vi "serpenbot_DDPG_learing_parallel.vi"() -> ()   [LabVIEW 2020]
uses:
  <vilib>/Analysis/Matrix/Datatypes/RealMatrix.ctl
  <vilib>/Analysis/Matrix/NI_Matrix.lvlib
  <vilib>/Analysis/NI_AALBase.lvlib
  <vilib>/Analysis/baseanly.llb/Real A x B.vi
  <vilib>/Analysis/NI_AALPro.lvlib
  <vilib>/Analysis/Matrix/Numeric/Conversions/Array To Matrix - RA.vi
  <vilib>/Analysis/Matrix/Numeric/Subtract/Subtract - RM,RM.vi
  <vilib>/Analysis/_algsub.llb/Real PseudoInverse Matrix.vi
panel:
  out "error out Y":errorcluster
  out "error out X":errorcluster
  out "laser control value":dbl[](array[numeric])
  out "current y":dbl
  out "current x":dbl
  out "control_loop_time":u32
  in  "stop":bool
  in  "Logging":bool caption="Enable"
  in  "k":T1
  in  "Diode Current\nSetting":dbl=3.0
  in  "Laser Repetition\nFrequency":i32=50000
  in  "VISA resource name":refnum<visa-resource-name>="COM14"
  in  "baud rate (9600)":u32=9600
  out "error out":errorcluster
  out "Identification system 1":string
  out "Conn. axes system 1":string[](array[string])
  out "Identification system 2":string
  out "Conn. axes system  2":string[](array[string])
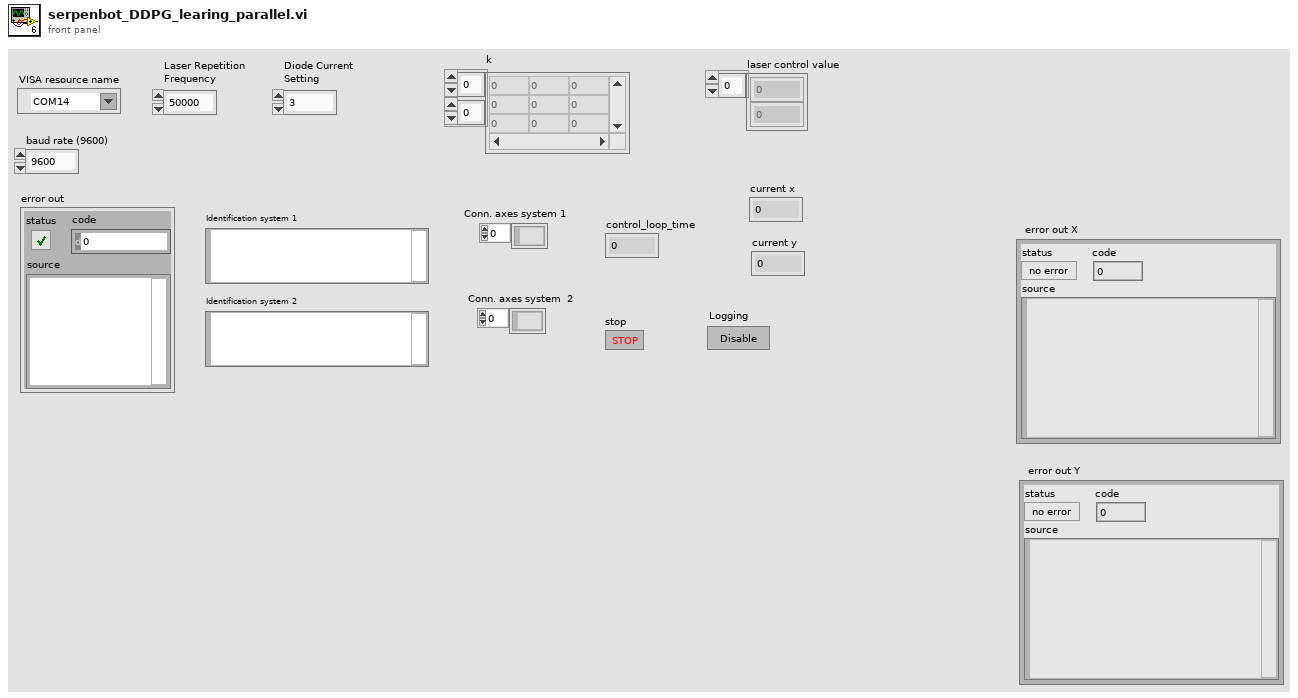
[diagram p1: front panel]
types:
  T1 = typedef "NI_Matrix.lvlib/RealMatrix.ctl" = dbl[][]
  T2 = cluster{"RS232 settings":cluster{"Portnumber":i32, "Baudrate":u16}, "USB settings":cluster{"S/N":string, "USB Search?":bool}, "TCP/IP settings":cluster{"Host address/name":string, "Port":i32, "Board":i32, "TCP/IP Search?":bool}}
  T3 = cluster{"Check FRF?":bool, "Referencing mode":enum16{"FRF (-> FNL)", "FRF", "FNL", "FPL", "RON OFF"}[]}
  T4 = cluster{"Force?":bool, "Dialog?":bool, "Stages":string[]}
  T5 = cluster{"Position":cluster{"x":sgl, "y":sgl}, "Angle":sgl, "Scale":sgl, "Score":sgl, "Bounding Box":cluster{"x":sgl, "y":sgl}[]}[]
  T6 = cluster{"[0]":cluster{"Position":cluster{"x":sgl, "y":sgl}, "Angle":sgl, "Scale":sgl, "Score":sgl, "Bounding Box":cluster{"x":sgl, "y":sgl}[]}, "[1]":cluster{"Position":cluster{"x":sgl, "y":sgl}, "Angle":sgl, "Scale":sgl, "Score":sgl, "Bounding Box":cluster{"x":sgl, "y":sgl}[]}, "[2]":cluster{"Position":cluster{"x":sgl, "y":sgl}, "Angle":sgl, "Scale":sgl, "Score":sgl, "Bounding Box":cluster{"x":sgl, "y":sgl}[]}, "[3]":cluster{"Position":cluster{"x":sgl, "y":sgl}, "Angle":sgl, "Scale":sgl, "Score":sgl, "Bounding Box":cluster{"x":sgl, "y":sgl}[]}, "[4]":cluster{"Position":cluster{"x":sgl, "y":sgl}, "Angle":sgl, "Scale":sgl, "Score":sgl, "Bounding Box":cluster{"x":sgl, "y":sgl}[]}, "[5]":cluster{"Position":cluster{"x":sgl, "y":sgl}, "Angle":sgl, "Scale":sgl, "Score":sgl, "Bounding Box":cluster{"x":sgl, "y":sgl}[]}, "[6]":cluster{"Position":cluster{"x":sgl, "y":sgl}, "Angle":sgl, "Scale":sgl, "Score":sgl, "Bounding Box":cluster{"x":sgl, "y":sgl}[]}, "[7]":cluster{"Position":cluster{"x":sgl, "y":sgl}, "Angle":sgl, "Scale":sgl, "Score":sgl, "Bounding Box":cluster{"x":sgl, "y":sgl}[]}, "[8]":cluster{"Position":cluster{"x":sgl, "y":sgl}, "Angle":sgl, "Scale":sgl, "Score":sgl, "Bounding Box":cluster{"x":sgl, "y":sgl}[]}}
  T7 = cluster{"Position":cluster{"x":sgl, "y":sgl}, "Angle":sgl, "Scale":sgl, "Score":sgl, "Bounding Box":cluster{"x":sgl, "y":sgl}[]}
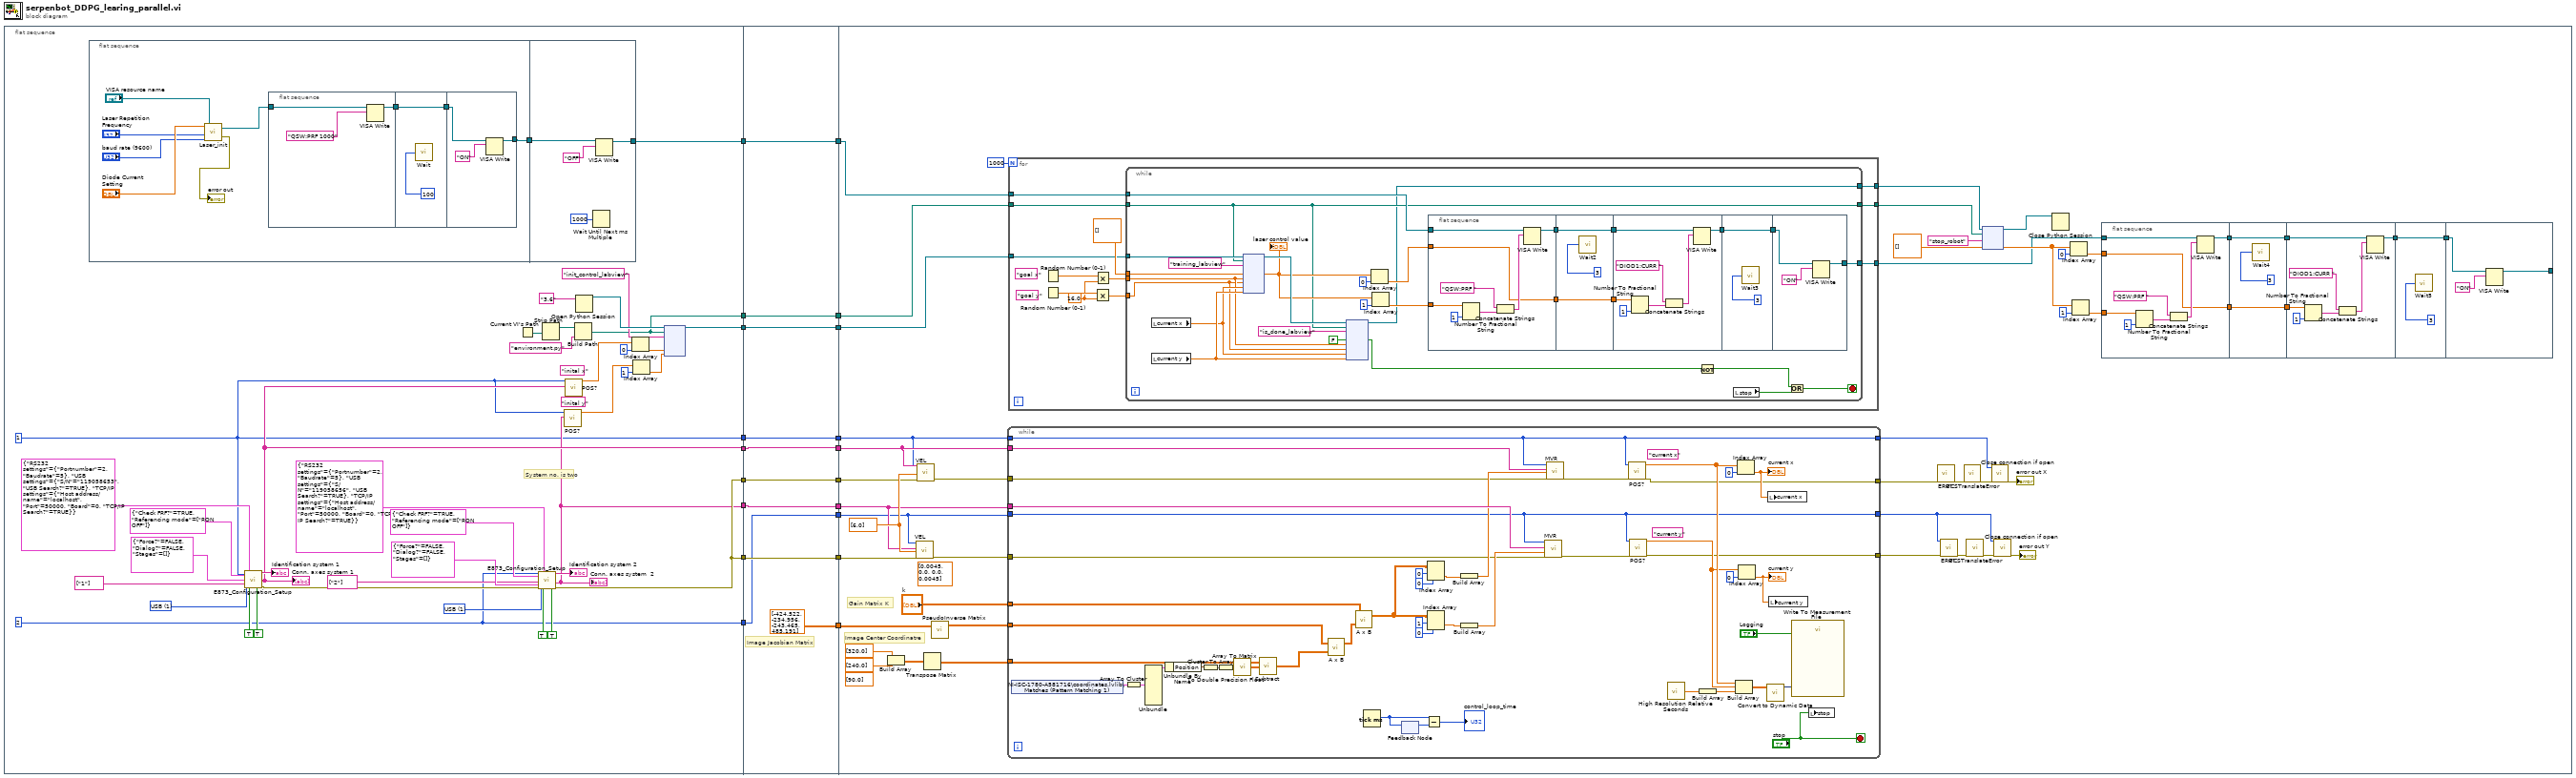
[diagram p0: block diagram]
diagram:
  n1 = flat-sequence {
    tunnel: [w56] -> w19
    tunnel: [w26] -> w18
    tunnel: [w28] -> w17
    tunnel: [w37] -> w16
    tunnel: [w27] -> w15
    tunnel: [w38] -> w14
    tunnel: [w37] -> w13
    tunnel: [w30] -> w12
    tunnel: [w29] -> w11
    tunnel: w19 -> [w88]
    tunnel: [w88] -> w10
    tunnel: w18 -> [w87]
    tunnel: w17 -> [w86]
    tunnel: w16 -> [w85]
    tunnel: w15 -> [w84]
    tunnel: w14 -> [w82]
    tunnel: [w87] -> w9
    tunnel: [w86] -> w8
    tunnel: [w85] -> w7
    tunnel: [w84] -> w6
    tunnel: w13 -> [w83]
    tunnel: [w83] -> w5
    tunnel: [w82] -> w4
    tunnel: [T1 [[-424.522, -234.956], [-243.465, 485.191]] ("J_init 2")] -> w3
    tunnel: w12 -> [w80]
    tunnel: w11 -> [w79]
    tunnel: [w80] -> w2
    tunnel: [w79] -> w1
    tunnel: w10 -> [w103]
    tunnel: w9 -> [w121]
    tunnel: w8 -> [w128]
    tunnel: w7 -> [w131]
    tunnel: w6 -> [w126]
    tunnel: w5 -> [w130]
    tunnel: w4 -> [w120]
    tunnel: w3 -> [w129]
    tunnel: w2 -> [w105]
    tunnel: w1 -> [w104]
    frame #0 {
      (unwired) "inital y"
      (unwired) "inital x"
      w41 = u16 1 items=["RS232", "USB", "TCP/IP"] ("Interface")
      w44 = u16 1 items=["RS232", "USB", "TCP/IP"] ("Interface")
      w38 = 2 ("System no.")
      w26 = 1 ("System no.")
      # "System no. is two"
      n2 = flat-sequence {
        tunnel: [w58] -> w57
        tunnel: w57 -> [w76]
        tunnel: [w75] -> w56
        frame #0 {
          n3 = call "Laser_init.vi"("baud rate (9600)"="baud rate (9600)", "Laser Repetition\nFrequency"="Laser Repetition\nFrequency", "VISA resource name"="VISA resource name", "Diode Current\nSetting"="Diode Current\nSetting") -> ("error out"=→"error out":errorcluster, "VISA Refnum out"=w59:refnum<visa-resource-name>)
          n4 = flat-sequence {
            tunnel: w59 -> [w69]
            tunnel: [w68] -> w66
            tunnel: w66 -> [w71]
            tunnel: [w71] -> w65
            tunnel: w65 -> [w72]
            tunnel: [w73] -> w58
            frame #0 {
              n5 = VISA Write(VISA resource name=w69, write buffer="QSW:PRF 1000" ("string")) -> (VISA resource name out=w68:refnum<visa-resource-name>)  [unwired: 1 in, 2 out]
            }
            frame #1 {
              n6 = call "Wait"("Count(mSec)"=u32 100) -> ()  [unwired: 1 out]
            }
            frame #2 {
              n7 = VISA Write(VISA resource name=w72, write buffer="ON") -> (VISA resource name out=w73:refnum<visa-resource-name>)  [unwired: 1 in, 2 out]
            }
          }
        }
        frame #1 {
          n8 = Wait Until Next ms Multiple(millisecond multiple=u32 1000) -> ()  [unwired: 1 out]
          n9 = VISA Write(VISA resource name=w76, write buffer="OFF") -> (VISA resource name out=w75:refnum<visa-resource-name>)  [unwired: 1 in, 2 out]
        }
      }
      n10 = call "E873_Configuration_Setup.vi"("System no."=w26, "Referencing"=T3 {"Check FRF?"=TRUE, "Referencing mode"=[enum."RON OFF"]}, "Interface"=w44, "All axes?"=TRUE, "Axes to move"=string[] ["1"], "Interface settings"=T2 {"RS232 settings"={"Portnumber"=2, "Baudrate"=5}, "USB settings"={"S/N"="119058653", "USB Search?"=TRUE}, "TCP/IP settings"={"Host address/name"="localhost", "Port"=50000, "Board"=0, "TCP/IP Search?"=TRUE}}, "Stage selection"=T4 {"Force?"=FALSE, "Dialog?"=FALSE, "Stages"=[]}, "Switch servo on?"=TRUE ("Use dialog to define\nconnected stages?")) -> ("Identification"=→"Identification system 1":string, "Conn. \nAxes"=w28:string[], "error out"=w53:errorcluster)  [unwired: 4 in, 5 out]
      "Conn. axes system 1" <- w28
      n11 = Current VI's Path() -> (path=w36:path)
      n12 = call "E873_Configuration_Setup.vi"("System no."=w38, "Referencing"=T3 {"Check FRF?"=TRUE, "Referencing mode"=[enum."RON OFF"]}, "Interface"=w41, "All axes?"=TRUE, "Axes to move"=string[] ["2"], "error in"=w53, "Interface settings"=T2 {"RS232 settings"={"Portnumber"=2, "Baudrate"=5}, "USB settings"={"S/N"="119058656", "USB Search?"=TRUE}, "TCP/IP settings"={"Host address/name"="localhost", "Port"=50000, "Board"=0, "TCP/IP Search?"=TRUE}}, "Stage selection"=T4 {"Force?"=FALSE, "Dialog?"=FALSE, "Stages"=[]}, "Switch servo on?"=TRUE ("Use dialog to define\nconnected stages?")) -> ("Identification"=→"Identification system 2":string, "Conn. \nAxes"=w27:string[], "error out"=w37:errorcluster)  [unwired: 3 in, 5 out]
      "Conn. axes system  2" <- w27
      n13 = Strip Path(path=w36) -> (stripped path=w35:path)  [unwired: 1 out]
      n14 = call "POS?.vi"("System no."=w26, "Axes to query"=w27) -> ("Position"=w20:dbl[])  [unwired: 3 in, 14 out]
      n15 = call "POS?.vi"("System no."=w26, "Axes to query"=w28) -> ("Position"=w23:dbl[])  [unwired: 3 in, 14 out]
      n16 = Build Path(base path=w35, name or relative path="environment.py") -> (appended path=w30:path)
      n17 = Open Python Session(python version="3.6" ("Python version")) -> (session out=w32:refnum<k35>)  [unwired: 2 in, 1 out]
      n18 = Index Array(array=w23, index=0) -> (element=w24:dbl)
      n19 = Index Array(array=w20, index=1) -> (element=w21:dbl)
      n20 = node(w32, w30, "init_control_labview" ("function name"), w24, w21) -> (w29:refnum<k35>)  [unwired: 5 in, 3 out]
    }
    frame #1 {
      # "Image Jacobian Matrix"
    }
    frame #2 {
      w132 = dbl[] [6.0] ("Velocity values")
      (unwired) T1 [[0.0045, 0.0], [0.0, 0.0045]] ("J_init 2")
      (unwired) dbl[] [90.0] ("element")
      # "Gain Matrix K"
      # "Image Center Coordinatre"
      n21 = Build Array(dbl[] [320.0] ("element"), dbl[] [240.0] ("element")) -> (w133:T1)
      n22 = call "VEL.vi"("System no."=w120, "Axes to set"=w126, "Velocity values"=w132, "error in"=w130) -> ("error out"=w125:errorcluster)  [unwired: 2 in, 13 out]
      n23 = call "VEL.vi"("System no."=w121, "Axes to set"=w128, "Velocity values"=w132, "error in"=w131) -> ("error out"=w127:errorcluster)  [unwired: 2 in, 13 out]
      n24 = Transpose Matrix(1:w133) -> (0:w122:T1)
      n25 = call-poly <vilib>:"PseudoInverse Matrix.vi"("Input Matrix"=w129) -> ("PseudoInverse Matrix"=w123:T1)  [unwired: 1 in, 1 out]
      n26 = while {
        tunnel: w125 -> [w227]
        tunnel: w120 -> [w201]
        tunnel: w126 -> [w245]
        tunnel: w127 -> [w228]
        tunnel: w128 -> [w244]
        tunnel: w121 -> [w203]
        tunnel: w123 -> [w233]
        tunnel: "k" -> [w232]
        tunnel: w122 -> [w231]
        tunnel: [w203] -> w92
        tunnel: [w202] -> w91
        tunnel: [w201] -> w90
        tunnel: [w200] -> w89
        stop <- "stop" stop-if-true
        (unwired) "current y"
        (unwired) "current x"
        n27 = shared-variable "NI-ISC-1780-A581716\\coordinates.lvlib\\Matches (Pattern Matching 1)"() -> (w220:T5)  [unwired: 1 in, 1 out]
        n28 = Array To Cluster(array=w220) -> (cluster=w221:T6)
        n29 = Unbundle(w221) -> ("[0]"=w222:T7)  [unwired: 8 out]
        n30 = Unbundle By Name(w222) -> ("Position"=w223:cluster{"x":sgl, "y":sgl})
        n31 = Cluster To Array(cluster=w223) -> (array=w224:sgl[])
        n32 = To Double Precision Float(number=w224) -> (double precision float=w225:dbl[])
        n33 = call-poly <vilib>:"Array To Matrix.vi"("Real 1D Array"=w225) -> ("Real Matrix (Column Vector)"=w219:T1)
        n34 = call-poly <vilib>:"Subtract.vi"("Real Matrix B"=w219, "Real Matrix A"=w231) -> ("A - B"=w239:T1)
        n35 = call-poly <vilib>:"A x B.vi"("B"=w239, "A"=w233) -> ("A x B"=w237:T1)  [unwired: 1 out]
        n36 = call-poly <vilib>:"A x B.vi"("B"=w237, "A"=w232) -> ("A x B"=w238:T1)  [unwired: 1 out]
        n37 = Tick Count (ms)() -> (millisecond timer value=w211:u32)
        n38 = feedback #1() -> (w234:u32)  [unwired: 1 in]
        n39 = feedback-in #1(w211) -> ()
        n40 = Subtract(x=w211, y=w234) -> (x-y=→"control_loop_time":u32)
        n41 = Index Array(array=w238, index (row)=0, index (col)=0) -> (element=w230:dbl)
        n42 = Index Array(array=w238, index (row)=1, index (col)=0) -> (element=w229:dbl)
        n43 = Build Array(w230) -> (w236:dbl[])
        n44 = Build Array(w229) -> (w235:dbl[])
        n45 = call "MVR.vi"("System no."=w201, "Axes to move"=w245, "Position values"=w235, "error in"=w227) -> ("error out"=w212:errorcluster)  [unwired: 1 in, 14 out]
        n46 = call "MVR.vi"("System no."=w203, "Axes to move"=w244, "Position values"=w236, "error in"=w228) -> ("error out"=w213:errorcluster)  [unwired: 1 in, 14 out]
        n47 = call "POS?.vi"("System no."=w203, "error in"=w213) -> ("Position"=w210:dbl[], "error out"=w202:errorcluster)  [unwired: 3 in, 13 out]
        n48 = call "POS?.vi"("System no."=w201, "error in"=w212) -> ("Position"=w208:dbl[], "error out"=w200:errorcluster)  [unwired: 3 in, 13 out]
        n49 = call <vilib>:"High Resolution Relative Seconds.vi"() -> ("relative seconds"=w215:dbl)
        n50 = Build Array(w215) -> (w214:dbl[])
        n51 = Build Array(w210, w208, w214) -> (w217:dbl[][])
        n52 = Index Array(array=w210, index=0) -> (element=w206:dbl)
        "current x" <- w206
        n53 = Index Array(array=w208, index=0) -> (element=w205:dbl)
        "current y" <- w205
        n54 = call "Convert to Dynamic Data"("2D Array"=w217) -> ("Dynamic Data Type"=w216:dynamicdata)  [unwired: 3 in]
        n55 = local write "current x"(w206) -> ()
        n56 = local write "current y"(w205) -> ()
        n57 = call "Write To Measurement File"("Signals"=w216, "Enable"="Logging") -> ()  [unwired: 15 in, 3 out]
        n58 = local write "stop"("stop") -> ()
      }
      n59 = for {
        N: 1000 -> [_]
        tunnel: w105 -> [w141]
        tunnel: w104 -> [w140]
        tunnel: w103 -> [w139]
        tunnel: [w138] -> w101
        tunnel: [w137] -> w100
        tunnel: [w136] -> w99
        w145 = 16.0
        (unwired) "goal y"
        (unwired) "goal x"
        n60 = Random Number (0-1)() -> (number: 0 to 1=w147:dbl)
        n61 = Random Number (0-1)() -> (number: 0 to 1=w146:dbl)
        n62 = Multiply(x=w146, y=w145) -> (x*y=w142:dbl)
        n63 = Multiply(x=w147, y=w145) -> (x*y=w143:dbl)
        n64 = while {
          tunnel: dbl[] [] -> [w161]
          tunnel: w143 -> [w158]
          tunnel: w142 -> [w157]
          tunnel: w141 -> [w154]
          tunnel: w140 -> [w156]
          tunnel: w139 -> [w155]
          tunnel: [w154] -> w138
          tunnel: [w153] -> w137
          tunnel: [w148] -> w136
          stop <- w151 stop-if-true
          n65 = local read "current x"() -> (w159:dbl)
          n66 = local read "current y"() -> (w160:dbl)
          n67 = node(w156, w154, "training_labview" ("function name"), w161, w158, w157, w159, w160) -> (w169:refnum<k35>, w163:dbl[])  [unwired: 5 in, 3 out]
          "laser control value" <- w163
          n68 = node(w169, w154, "is_done_labview" ("function name"), FALSE, w158, w157, w159, w160) -> (w153:refnum<k35>, w149:bool)  [unwired: 5 in, 3 out]
          n69 = Index Array(array=w163, index=0) -> (element=w166:dbl)
          n70 = Index Array(array=w163, index=1) -> (element=w162:dbl)
          n71 = flat-sequence {
            tunnel: w155 -> [w180]
            tunnel: [w179] -> w176
            tunnel: w162 -> [w178]
            tunnel: w166 -> [w177]
            tunnel: [w177] -> w175
            tunnel: [w187] -> w174
            tunnel: [w185] -> w173
            tunnel: w176 -> [w187]
            tunnel: w175 -> [w185]
            tunnel: [w194] -> w172
            tunnel: w174 -> [w192]
            tunnel: w173 -> [w189]
            tunnel: w172 -> [w196]
            tunnel: [w196] -> w171
            tunnel: w171 -> [w198]
            tunnel: [w197] -> w148
            frame #0 {
              n72 = Number To Fractional String(number=w178, precision (6)=i16 1) -> (F-format string=w183:string)  [unwired: 2 in]
              n73 = Concatenate Strings("QSW:PRF " ("string"), w183) -> (w184:string)
              n74 = VISA Write(VISA resource name=w180, write buffer=w184) -> (VISA resource name out=w179:refnum<visa-resource-name>)  [unwired: 1 in, 2 out]
            }
            frame #1 {
              n75 = call "Wait2"("Count(mSec)"=u32 3) -> ()  [unwired: 1 out]
            }
            frame #2 {
              n76 = Number To Fractional String(number=w189, precision (6)=i16 1) -> (F-format string=w190:string)  [unwired: 2 in]
              n77 = Concatenate Strings("DIOD1:CURR " ("string"), w190) -> (w193:string)
              n78 = VISA Write(VISA resource name=w192, write buffer=w193) -> (VISA resource name out=w194:refnum<visa-resource-name>)  [unwired: 1 in, 2 out]
            }
            frame #3 {
              n79 = call "Wait3"("Count(mSec)"=u32 3) -> ()  [unwired: 1 out]
            }
            frame #4 {
              n80 = VISA Write(VISA resource name=w198, write buffer="ON") -> (VISA resource name out=w197:refnum<visa-resource-name>)  [unwired: 1 in, 2 out]
            }
          }
          n81 = Not(x=w149) -> (.not. x?=w150:bool)
          n82 = local read "stop"() -> (w152:bool)
          n83 = Or(x=w150, y=w152) -> (x .or. y?=w151:bool)
        }
      }
      n84 = call "ERR?.vi"("error in"=w91) -> ("error out"=w96:errorcluster)  [unwired: 1 in, 17 out]
      n85 = call "ERR?.vi"("System no."=w90, "error in"=w89) -> ("error out"=w93:errorcluster)  [unwired: 17 out]
      n86 = call "GCSTranslateError.vi"("error in"=w96) -> ("error out"=w97:errorcluster)  [unwired: 18 out]
      n87 = call "GCSTranslateError.vi"("error in"=w93) -> ("error out"=w94:errorcluster)  [unwired: 18 out]
      n88 = node(w100, w101, "stop_robot" ("function name"), dbl[] []) -> (w111:refnum<k35>, w106:dbl[])  [unwired: 1 in, 3 out]
      n89 = call "Close connection if open.vi"("System no."=w92, "error in"=w97) -> ("error out"=→"error out X":errorcluster)  [unwired: 1 in, 16 out]
      n90 = call "Close connection if open.vi"("System no."=w90, "error in"=w94) -> ("error out"=→"error out Y":errorcluster)  [unwired: 1 in, 16 out]
      n91 = Close Python Session(session in=w111) -> ()  [unwired: 1 in, 1 out]
      n92 = Index Array(array=w106, index=0) -> (element=w108:dbl)
      n93 = Index Array(array=w106, index=1) -> (element=w107:dbl)
      n94 = flat-sequence {
        tunnel: w99 -> [w249]
        tunnel: [w248] -> w119
        tunnel: w107 -> [w247]
        tunnel: w108 -> [w246]
        tunnel: [w246] -> w118
        tunnel: [w256] -> w117
        tunnel: [w254] -> w116
        tunnel: w119 -> [w256]
        tunnel: w118 -> [w254]
        tunnel: [w263] -> w115
        tunnel: w117 -> [w261]
        tunnel: w116 -> [w258]
        tunnel: w115 -> [w265]
        tunnel: [w265] -> w114
        tunnel: w114 -> [w267]
        tunnel: [w266] -> _
        frame #0 {
          n95 = Number To Fractional String(number=w247, precision (6)=i16 1) -> (F-format string=w252:string)  [unwired: 2 in]
          n96 = Concatenate Strings("QSW:PRF " ("string"), w252) -> (w253:string)
          n97 = VISA Write(VISA resource name=w249, write buffer=w253) -> (VISA resource name out=w248:refnum<visa-resource-name>)  [unwired: 1 in, 2 out]
        }
        frame #1 {
          n98 = call "Wait4"("Count(mSec)"=u32 3) -> ()  [unwired: 1 out]
        }
        frame #2 {
          n99 = Number To Fractional String(number=w258, precision (6)=i16 1) -> (F-format string=w259:string)  [unwired: 2 in]
          n100 = Concatenate Strings("DIOD1:CURR " ("string"), w259) -> (w262:string)
          n101 = VISA Write(VISA resource name=w261, write buffer=w262) -> (VISA resource name out=w263:refnum<visa-resource-name>)  [unwired: 1 in, 2 out]
        }
        frame #3 {
          n102 = call "Wait5"("Count(mSec)"=u32 3) -> ()  [unwired: 1 out]
        }
        frame #4 {
          n103 = VISA Write(VISA resource name=w267, write buffer="ON") -> (VISA resource name out=w266:refnum<visa-resource-name>)  [unwired: 1 in, 2 out]
        }
      }
    }
  }
